vi "LVClass_WavefrontCorrector Get Actuator Current Position.vi"(0 "WavefrontCorrector in":refnum<class "WavefrontCorrector.lvclass">, 5 "Index of actuator":i32, 11 "error in (no error)":errorcluster) -> (4 "WavefrontCorrector out":refnum<class "WavefrontCorrector.lvclass">, 6 "Position":i32, 15 "error out":errorcluster)   [LabVIEW 2020, in "WavefrontCorrector.lvclass"]
uses:
  WavefrontCorrector.lvclass
  WavefrontCorrector.lvclass/WavefrontCorrector.ctl
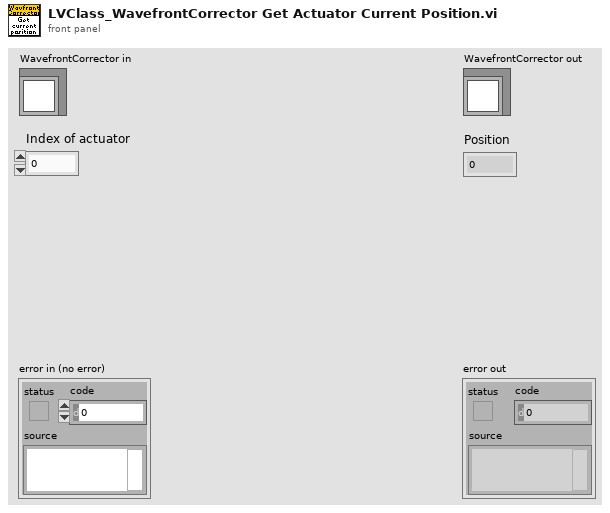
[diagram p1: front panel]
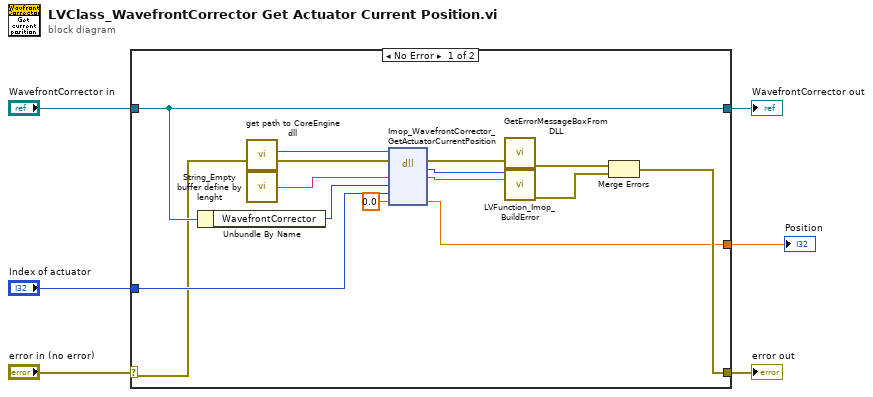
[diagram p0: block diagram]
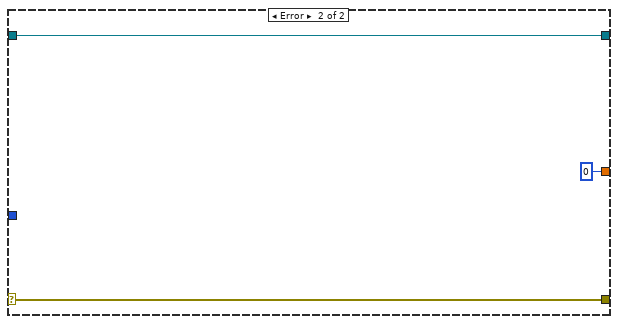
[diagram p2: hidden frame]
diagram:
  n1 = case shown="No Error" "error in (no error)" {
    selector: "error in (no error)" -> [w9 w23]
    tunnel: [w10 w23] -> w5
    tunnel: [w18 w22] -> w3
    tunnel: "WavefrontCorrector in" -> [w18 w22]
    tunnel: "Index of actuator" -> [w16 _]
    tunnel: [w8 0 ("Position")] -> w1
    frame No Error {
      n2 = Unbundle By Name(w18) -> ("WavefrontCorrector"=w17:i32)
      n3 = call "get path to CoreEngine dll.vi"() -> ("path to c_interface_vc100.dll"=w20:path)  [unwired: 12 in, 3 out]
      n4 = call "String_Empty buffer define by lenght.vi"() -> ("Empty buffer"=w19:string)  [unwired: 1 in]
      n5 = dll-call lib="D:/FLE/0.Code/CoreEngine4_Suite/LV2011_interface/DLLs/c_interface_vc100.dll" fn="Imop_WavefrontCorrector_GetActuatorCurrentPosition"(path in=w20, error in=w9, "Message"=w19, "WavefrontCorrector"=w17, "Index of actuator"=w16, "Position"=sgl 0.0) -> (error out=w15:errorcluster, "return type"=w13:i32, "Message"=w12:string, "Position"=w8:sgl)  [unwired: 3 in, 1 out]
      n6 = call "GetErrorMessageBoxFromDLL.vi"("error IN"=w15) -> ("error OUT"=w14:errorcluster)  [unwired: 10 in]
      n7 = call "LVFunction_Imop_BuildError.vi"("code"=w13, "String to Prepend to source (\"\")"=w12) -> ("error out"=w11:errorcluster)  [unwired: 13 in]
      n8 = Merge Errors(w14, w11) -> (w10:errorcluster)
    }
    frame Error {
    }
  }
  "error out" <- w5
  "WavefrontCorrector out" <- w3
  "Position" <- w1
